vi "PumpValve.vi"() -> ()   [LabVIEW 2015]
uses:
  <vilib>/DAQmx/write.llb/DAQmx Write (Digital 1D Bool NChan 1Samp 1Line).vi
  <vilib>/DAQmx/miscellaneous.llb/DAQmx Fill In Error Info.vi
panel:
  in  "stop":bool
  in  "Drain":bool
  in  "Fill":bool
  in  "Pump 2":bool
  in  "Blue Valve":bool
  in  "Green Valve":bool
  out "Green":i32
  out "Blue":i32
  out "Pump":i32
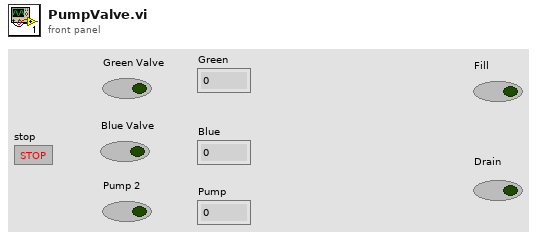
[diagram p1: front panel]
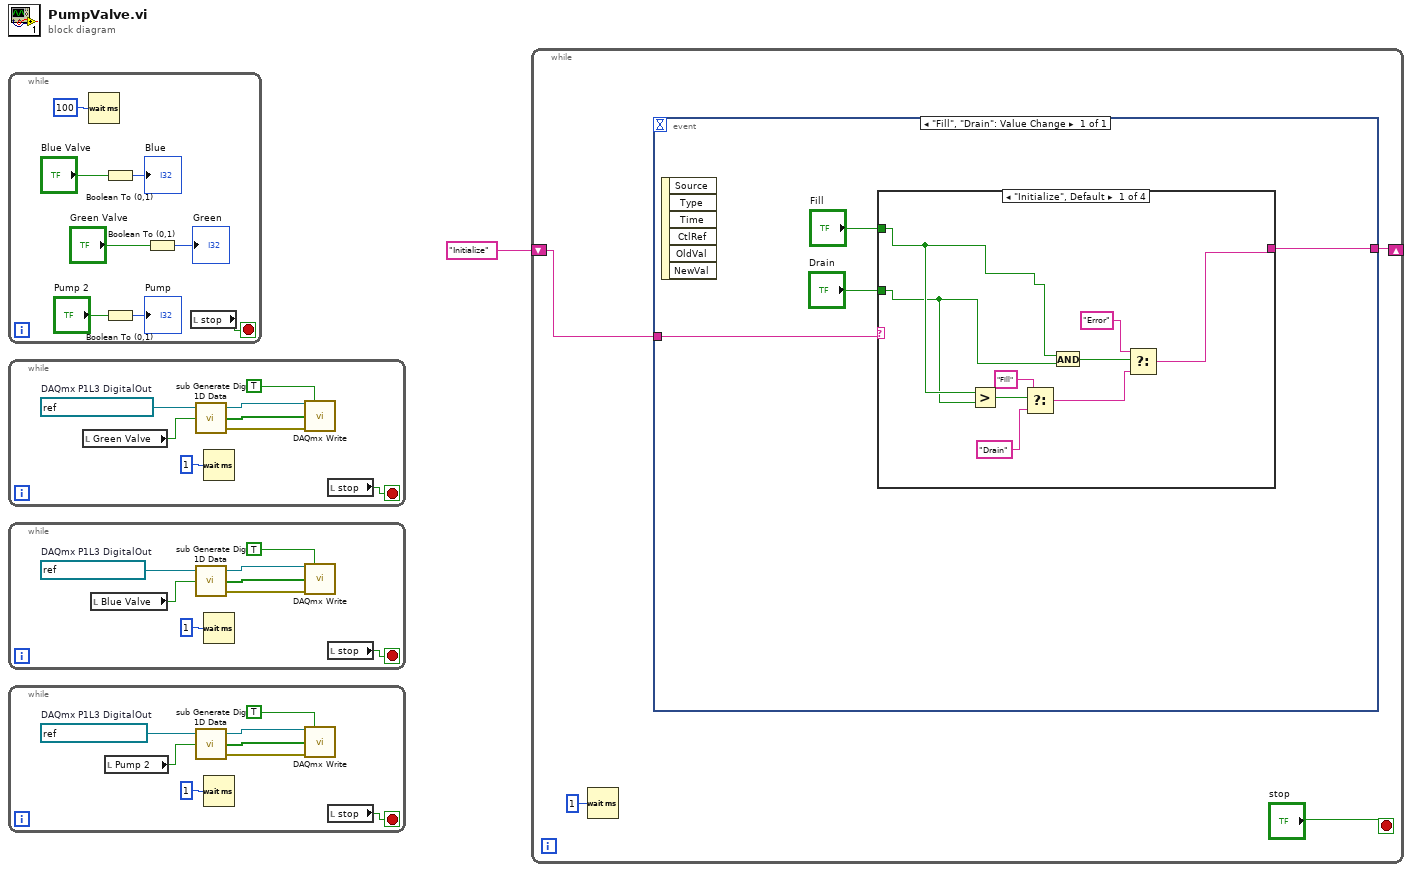
[diagram p0: block diagram]
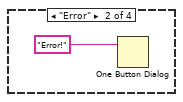
[diagram p2: hidden frame]
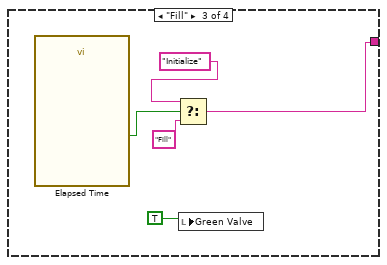
[diagram p3: hidden frame]
diagram:
  n1 = while {
    stop <- w2 stop-if-true
    n2 = Wait (ms)(milliseconds to wait=u32 100) -> ()  [unwired: 1 out]
    n3 = Boolean To (0,1)(Boolean="Blue Valve") -> (0, 1=→"Blue":i16)
    n4 = Boolean To (0,1)(Boolean="Pump 2") -> (0, 1=→"Pump":i16)
    n5 = Boolean To (0,1)(Boolean="Green Valve") -> (0, 1=→"Green":i16)
    n6 = local read "stop"() -> (w2:bool)
  }
  n7 = while {
    stop <- w10 stop-if-true
    w17 = refnum<k21> "DigitalOutGreen"  # DAQmx P1L3 DigitalOut
    n8 = local read "Green Valve"() -> (w11:bool)
    n9 = call <vilib>:"sub Generate Dig 1D Data.vi"("initial value"=w11, "task in"=w17) -> ("error out"=w14:errorcluster, "Data"=w15:bool[], "task out"=w16:refnum<k21>)  [unwired: 1 in]
    n10 = Wait (ms)(milliseconds to wait=u32 1) -> ()  [unwired: 1 out]
    n11 = call-poly <vilib>:"DAQmx Write.vi"("task/channels in"=w16, "auto start"=TRUE, "data"=w15, "error in"=w14) -> ()  [unwired: 9 in, 3 out]
    n12 = local read "stop"() -> (w10:bool)
  }
  n13 = while {
    stop <- w18 stop-if-true
    w25 = refnum<k21> "DigitalOutBlue"  # DAQmx P1L3 DigitalOut
    n14 = local read "Blue Valve"() -> (w19:bool)
    n15 = call <vilib>:"sub Generate Dig 1D Data.vi"("initial value"=w19, "task in"=w25) -> ("error out"=w22:errorcluster, "Data"=w23:bool[], "task out"=w24:refnum<k21>)  [unwired: 1 in]
    n16 = Wait (ms)(milliseconds to wait=u32 1) -> ()  [unwired: 1 out]
    n17 = call-poly <vilib>:"DAQmx Write.vi"("task/channels in"=w24, "auto start"=TRUE, "data"=w23, "error in"=w22) -> ()  [unwired: 9 in, 3 out]
    n18 = local read "stop"() -> (w18:bool)
  }
  n19 = while {
    stop <- w26 stop-if-true
    w33 = refnum<k21> "P0L0DigitalOut"  # DAQmx P1L3 DigitalOut
    n20 = local read "Pump 2"() -> (w27:bool)
    n21 = call <vilib>:"sub Generate Dig 1D Data.vi"("initial value"=w27, "task in"=w33) -> ("error out"=w30:errorcluster, "Data"=w31:bool[], "task out"=w32:refnum<k21>)  [unwired: 1 in]
    n22 = Wait (ms)(milliseconds to wait=u32 1) -> ()  [unwired: 1 out]
    n23 = call-poly <vilib>:"DAQmx Write.vi"("task/channels in"=w32, "auto start"=TRUE, "data"=w31, "error in"=w30) -> ()  [unwired: 9 in, 3 out]
    n24 = local read "stop"() -> (w26:bool)
  }
  n25 = while {
    shift-right: [w36] -> _
    shift-left: "Initialize" -> [w37]
    stop <- "stop" stop-if-true
    n26 = Wait (ms)(milliseconds to wait=u32 1) -> ()  [unwired: 1 out]
    n27 = event shown="[0] \"Fill\", \"Drain\": Value Change" {
      selector: _ -> [_]
      dyn-events: _ -> [_]
      timeout: _ -> [_]
      tunnel: w37 -> [w39]
      tunnel: [w38] -> w36
      event "Fill", "Drain": Value Change {
        n28 = event-data() -> ()  [unwired: 1 in, 6 out]
        n29 = case shown="\"Initialize\", Default" w39 {
          tunnel: "Fill" -> [w47 _ _ _]
          tunnel: "Drain" -> [w46 _ _ _]
          tunnel: [w48 _ w54 _] -> w38
          frame "Initialize", Default {
            n30 = Greater?(x=w47, y=w46) -> (0:w45:bool)
            n31 = Select(t="Fill", s=w45, f="Drain") -> (s? t:f=w44:string)
            n32 = And(x=w47, y=w46) -> (x .and. y?=w50:bool)
            n33 = Select(t="Error", s=w50, f=w44) -> (s? t:f=w48:string)
          }
          frame "Error" {
            n34 = One Button Dialog(message="Error!") -> ()  [unwired: 1 in, 1 out]
          }
          frame "Fill" {
            n35 = call "Elapsed Time"() -> ("Time has Elapsed"=w56:bool)  [unwired: 12 in, 7 out]
            n36 = Select(t="Initialize", s=w56, f="Fill") -> (s? t:f=w54:string)
            n37 = local write "Green Valve"(TRUE) -> ()
          }
          frame "Drain" {
          }
        }
      }
    }
  }
